vi "Write R_W_.vi"(8 "error in (no error)":errorcluster, 10 "R/W?":T1, 11 "SPI Root Pattern Creator in":refnum<class "SPI Root Pattern Creator.lvclass">) -> (0 "error out":errorcluster, 3 "SPI Root Pattern Creator out":refnum<class "SPI Root Pattern Creator.lvclass">)   [LabVIEW 2018, in "SPI Root Pattern Creator.lvlib" / "SPI Root Pattern Creator.lvclass"]
uses:
  SPI Root Pattern Creator.lvclass
  Ctls/RW Options.ctl
  SPI Root Pattern Creator.lvclass/SPI Root Pattern Creator.ctl
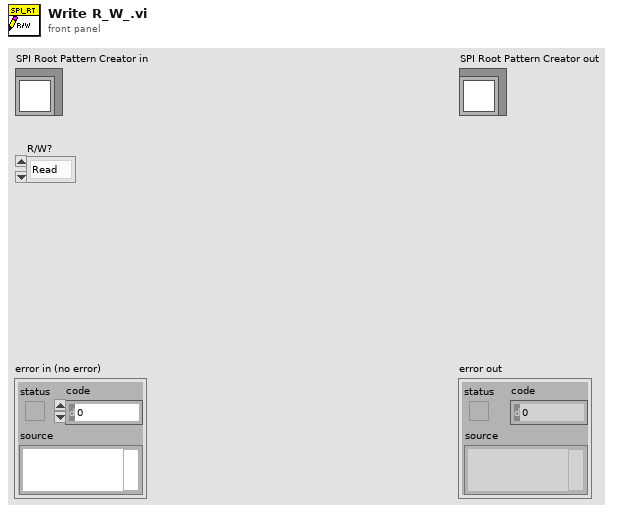
[diagram p1: front panel]
types:
  T1 = typedef "RW Options.ctl" = enum16{"Read", "Write", "R/W"}
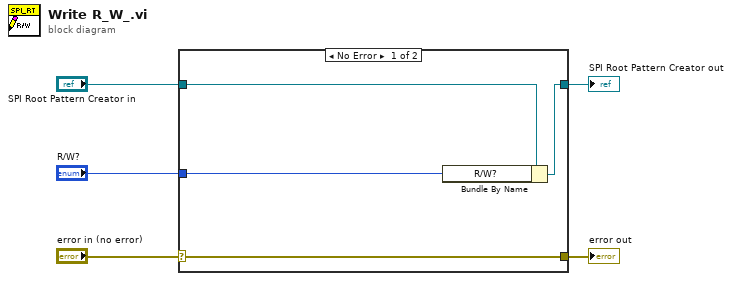
[diagram p0: block diagram]
diagram:
  n1 = case shown="No Error" "error in (no error)" {
    selector: "error in (no error)" -> [w9 w10]
    tunnel: [w9 w10] -> w4
    tunnel: [w7 w11] -> w2
    tunnel: "SPI Root Pattern Creator in" -> [w8 w11]
    tunnel: "R/W?" -> [w6 _]
    frame No Error {
      n2 = Bundle By Name(cluster=w8, "R/W?"=w6) -> (w7:refnum<class "SPI Root Pattern Creator.lvclass">)
    }
    frame Error {
    }
  }
  "error out" <- w4
  "SPI Root Pattern Creator out" <- w2
